vi "1B_AnalyzeAmplitudeRamp_Trim.vi"(8 "Array":waveform(dbl)[](array[waveform])=[{"t0"=timestamp(3464860426.1720004 s since 1904-01-01), "dt"=3.8400000000000005e-06, "Y"=array[16000 elements]}, {"t0"=timestamp(3464860427.2660003 s since 1904-01-01), "dt"=3.8400000000000005e-06, "Y"=array[16000 elements]}, {"t0"=timestamp(3464860428.3440003 s since 1904-01-01), "dt"=3.8400000000000005e-06, "Y"=array[16000 elements]}, {"t0"=timestamp(3464860429.453 s since 1904-01-01), "dt"=3.8400000000000005e-06, "Y"=array[16000 elements]}, {"t0"=timestamp(3464860430.563 s since 1904-01-01), "dt"=3.8400000000000005e-06, "Y"=array[16000 elements]}, {"t0"=timestamp(3464860431.6720004 s since 1904-01-01), "dt"=3.8400000000000005e-06, "Y"=array[16000 elements]}, {"t0"=timestamp(3464860432.766 s since 1904-01-01), "dt"=3.8400000000000005e-06, "Y"=array[16000 elements]}, {"t0"=timestamp(3464860433.8750005 s since 1904-01-01), "dt"=3.8400000000000005e-06, "Y"=array[16000 elements]}, {"t0"=timestamp(3464860434.9690003 s since 1904-01-01), "dt"=3.8400000000000005e-06, "Y"=array[16000 elements]}], 9 "Min time ( sec )":dbl=1.0, 10 "Max Time ( sec )":dbl=10.0, 11 "Elapsed time from Active Stim ( sec )":dbl[](array[numeric])=[1.8767312026320724, 2.978631206395221, 4.068465751042822, 5.166899951203959, 6.281533743458567, 7.396964385960018, 8.492272259914898, 9.593095214062487, 10.689171075006016] format="%#.1g") -> (0 "Array out":waveform(dbl)[](array[waveform])=[{"t0"=timestamp(3464860426.1720004 s since 1904-01-01), "dt"=3.8400000000000005e-06, "Y"=array[16000 elements]}, {"t0"=timestamp(3464860427.2660003 s since 1904-01-01), "dt"=3.8400000000000005e-06, "Y"=array[16000 elements]}, {"t0"=timestamp(3464860428.3440003 s since 1904-01-01), "dt"=3.8400000000000005e-06, "Y"=array[16000 elements]}, {"t0"=timestamp(3464860429.453 s since 1904-01-01), "dt"=3.8400000000000005e-06, "Y"=array[16000 elements]}, {"t0"=timestamp(3464860430.563 s since 1904-01-01), "dt"=3.8400000000000005e-06, "Y"=array[16000 elements]}, {"t0"=timestamp(3464860431.6720004 s since 1904-01-01), "dt"=3.8400000000000005e-06, "Y"=array[16000 elements]}, {"t0"=timestamp(3464860432.766 s since 1904-01-01), "dt"=3.8400000000000005e-06, "Y"=array[16000 elements]}, {"t0"=timestamp(3464860433.8750005 s since 1904-01-01), "dt"=3.8400000000000005e-06, "Y"=array[16000 elements]}, {"t0"=timestamp(3464860434.9690003 s since 1904-01-01), "dt"=3.8400000000000005e-06, "Y"=array[16000 elements]}], 3 "Elapsed time from Active Stim ( sec ) out":dbl[](array[numeric])=[1.8767312026320724, 2.978631206395221, 4.068465751042822, 5.166899951203959, 6.281533743458567, 7.396964385960018, 8.492272259914898, 9.593095214062487, 10.689171075006016] format="%#.1g")   [LabVIEW 2010]
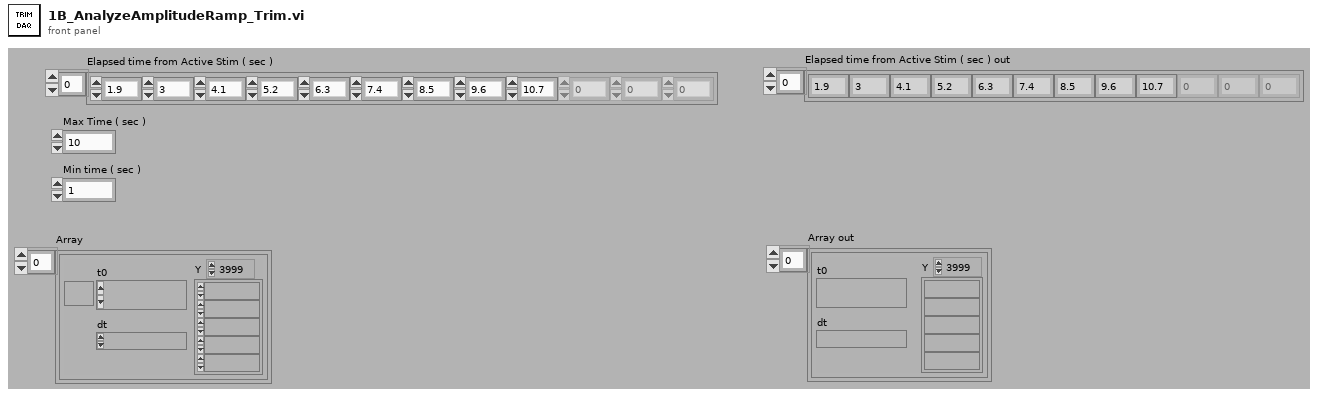
[diagram p1: front panel]
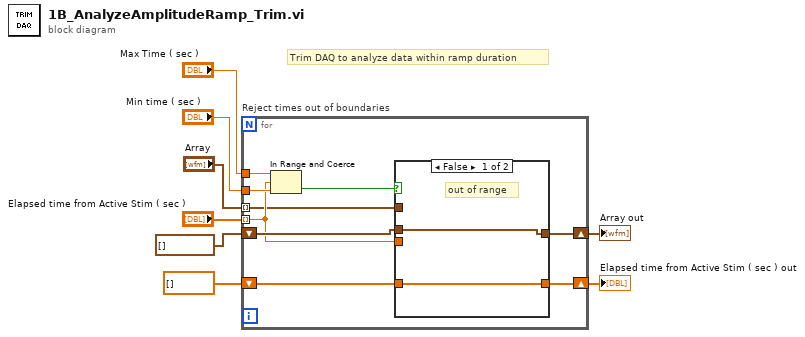
[diagram p0: block diagram]
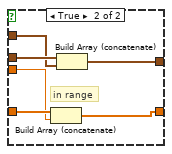
[diagram p2: hidden frame]
diagram:
  # "Trim DAQ to analyze data within ramp duration"
  n1 = for "Reject times out of boundaries" {
    shift-right: [w17] -> w8
    shift-left: waveform(dbl)[] [] ("Array out") -> [w13]
    tunnel: "Array" -> [w9] mode=indexing
    tunnel: "Elapsed time from Active Stim ( sec )" -> [w10] mode=indexing
    tunnel: "Max Time ( sec )" -> [w16]
    tunnel: "Min time ( sec )" -> [w15]
    shift-right: [w12] -> w2
    shift-left: dbl[] [] -> [w11]
    n2 = In Range and Coerce(upper limit=w16, x=w10, lower limit=w15) -> (In Range?=w14:bool)  [unwired: 1 out]
    n3 = case shown="False" w14 {
      tunnel: [w19 w25] -> w17
      tunnel: w13 -> [w19 w21]
      tunnel: [w18 w24] -> w12
      tunnel: w11 -> [w18 w23]
      tunnel: w10 -> [_ w22]
      tunnel: w9 -> [_ w20]
      frame False {
        # "out of range"
      }
      frame True {
        # "in range"
        n4 = Build Array (concatenate)(w23, w22) -> (w24:dbl[])
        n5 = Build Array (concatenate)(w21, w20) -> (w25:waveform(dbl)[])
      }
    }
  }
  "Elapsed time from Active Stim ( sec ) out" <- w2
  "Array out" <- w8
